vi "发送数值转字符串.vi"(10 "输入数据_U16":u16[](array[numeric]) format="%x") -> (2 "字符串":string)   [LabVIEW 2010]
panel:
  # "用于发送数值时将U16转为字符串"
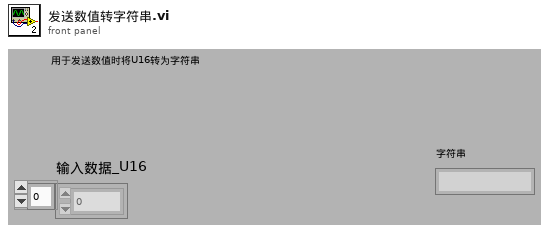
[diagram p1: front panel]
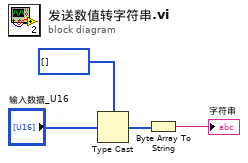
[diagram p0: block diagram]
diagram:
  n1 = Type Cast(type=u8[] [], x="输入数据_U16") -> (*(type *) &x=w1:u8[])
  n2 = Byte Array To String(unsigned byte array=w1) -> (string=→"字符串":string)
